vi "FPGA live imaging reset.vi"(8 "error in (no error)":errorcluster, 11 "FPGA VI Ref":T1) -> (0 "error out":errorcluster)   [LabVIEW 2013]
uses:
  RIG-SPECIFIC FILES/FPGA Refs/FPGA Ref.ctl
  <vilib>/rvi/interface/common/niFpgaWaitOnOcc.vi
  <vilib>/Utility/error.llb/Error Cluster From Error Code.vi
  <vilib>/rvi/errors/niLvFpgaAdjustHostInterfaceError.vi
  <vilib>/rvi/interface/nirviReadWriteControl/nirviReadWriteControl.xnode
  NiFpgaLv.dll
  <vilib>/rvi/interface/Simulation/niFpgaSimulationCallBeginRW.vi
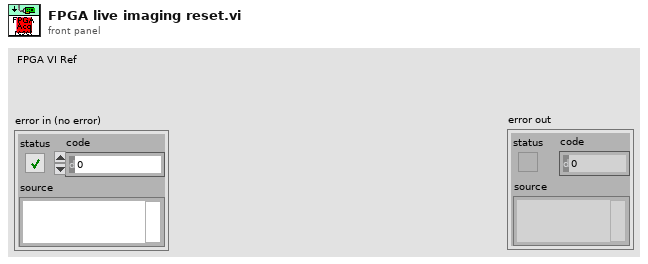
[diagram p1: front panel]
types:
  T1 = typedef "FPGA Ref.ctl" = refnum<k20>
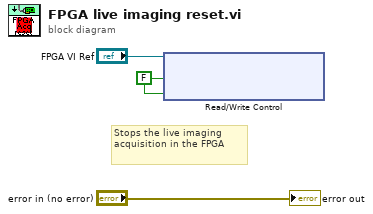
[diagram p0: block diagram]
diagram:
  w1 = FALSE ("live_scan")
  # "Stops the live imaging acquisition in the FPGA"
  n1 = xnode "Read/Write Control"("FPGA VI Reference In"="FPGA VI Ref", "live_scan"=w1, "live_scan (triggers module)"=w1) -> ()  [unwired: 1 in, 2 out]
  "error out" <- "error in (no error)"
